vi "RH_Auto_with_Lockin_clear_3.vi"() -> ()   [LabVIEW 2019]
uses:
  <vilib>/Instr/_visa.llb/VISA Configure Serial Port (Instr).vi
  <vilib>/ptbypt/NI_PtbyPt.lvlib
panel:
  out "T Graph":cluster{"X":dbl[], "Y":dbl[]}[](graph) caption="XY Graph"
  in  "Ramp [K/min]":bool
  in  "Ramp Mode":bool
  in  "Lakeshore Termination Character":u8=10 format="%.0x"
  in  "Apply voltage":bool
  out "read buffer":string
  in  "Target [V]":string
  in  "start [V]":string
  in  "Keithley2400":refnum<visa-resource-name>="GPIB1::15::INSTR"
  out "Resistance [Ohm]":dbl=97.3586 format="%#_6f"
  out "Lockin y (V)":dbl=136.05
  out "Lockin x (V)":dbl=0.000139774
  in  "On:Delta  Off:Lock-in":bool=TRUE
  in  "I for Lockin [A]":dbl=5e-06 format="%#_6e"
  out "Lockin Y (V)":dbl=-136.536
  out "Lockin X (V)":dbl=0.000486793
  in  "Lockin SR830":refnum<visa-resource-name>="GPIB1::8::INSTR"
  in  "Main sorb T control":bool
  in  "Wait [min]":i32
  in  "LakeShore335 (for He3)":refnum<visa-resource-name>="COM4"
  in  "Temp control off":bool
  out "Sample  T [K]":dbl=1.4
  out "Waiting T-stability":bool caption="stabilizing"
  in  "Set Initial Field":bool
  in  "Field [T]":dbl
  in  "Period [s]":dbl=0.3 caption="Delay Time (s)"
  in  "Measure R-T":bool
  in  "Save R-T":bool
  out "R-T":cluster{"X":dbl[], "Y":dbl[]}[](graph) caption="XY Graph"
  out "Rate [K/min]":dbl=-2.426094015917322 format="%#_6f"
  in  "Reset":bool
  in  "Stop":bool
  in  "Pause off":bool
  in  "Compliance [V]":dbl=1.0 format="%#_6f"
  out "R-H":cluster{"X":dbl[], "Y":dbl[]}[](graph) caption="XY Graph"
  in  "Reset":bool
  in  "Folder":path=path "C:/User Data/Graham" caption="Filename"
  out "Filename Out":path=path "C:/User Data/Bart/CG014_1012_3.00K"
  in  "File name":string="CG017a_3uA"
  out "VTI [K]":dbl=3.087
  out "VTI [K]":dbl=84.053
  out "Sample Temp [K]":dbl=1.4
  out "Magnetic Field [T]":dbl=2.97271
  out "Delta reading [Ohm]":dbl
  out "Delta Reading [Ohm]":dbl=355.153687
  out "Sample Temp [K]":dbl=186.475
  in  "Abort Delta":bool
  in  "Arm Delta":bool
  in  "DELAY [sec]":dbl=0.002 format="%#_6e"
  in  "I-HIGH [A]":dbl=1e-05 format="%#_6e"
  in  "Measure R-H":bool
  in  "Rate [K/min]":dbl=10.0
  in  "Set Temp [K]":dbl=20.0
  in  "Set Temperature":bool
  out "Magnetic Field [T]":dbl
  in  "Rate [T/min]":dbl=0.5
  in  "Set Field [T]":dbl
  in  "Set Field":bool
  in  "Keithley":refnum<visa-resource-name>="GPIB1::20::INSTR"
  in  "Skip":bool
  in  "Wait T-stable [min]":i32=30
  in  "period (s)":dbl=0.5 min=0.0 max=1111.0 step=0.1
  in  "stop 2":bool caption="Pause"
  in  "Wait field stable [sec]":dbl=20.0
  in  "Magnet Power supply":refnum<visa-resource-name>="COM6"
  in  "Set Field [T]   Rate [T/min]":dbl[][](array[numeric])=[[0.0, 0.2], [-6.0, 0.2], [0.0, 0.2], [6.0, 0.2]]
  in  "Set Temp [K]":dbl[][](array[numeric])=[[10.0, 5.0], [0.0, 5.0], [0.0, 5.0], [0.0, 5.0], [0.0, 5.0]]
  in  "LakeShore340":refnum<visa-resource-name>="COM7"
  out "error out 3":errorcluster={"status"=FALSE, "code"=1073676294, "source"="VISA Read in RH_Auto_with_Lockin_clear.vi"}
  # "Manual control"
  # "R-H Auto Measurement"
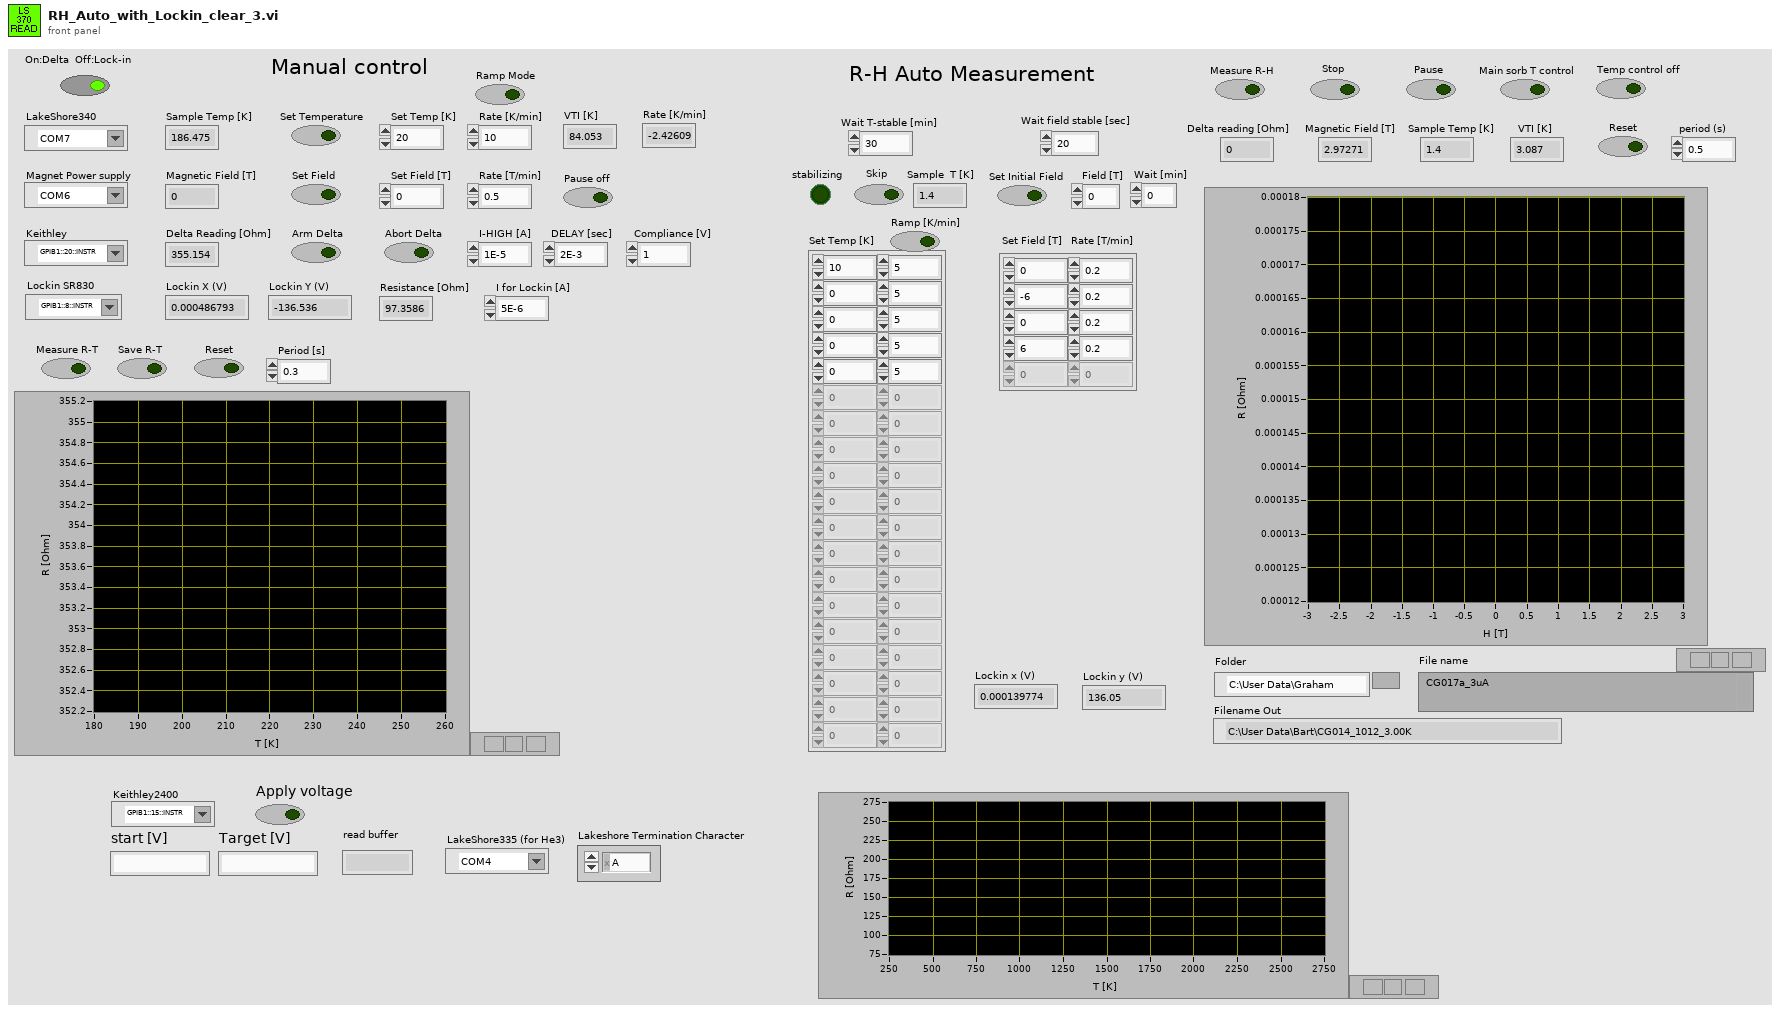
[diagram p1: front panel]
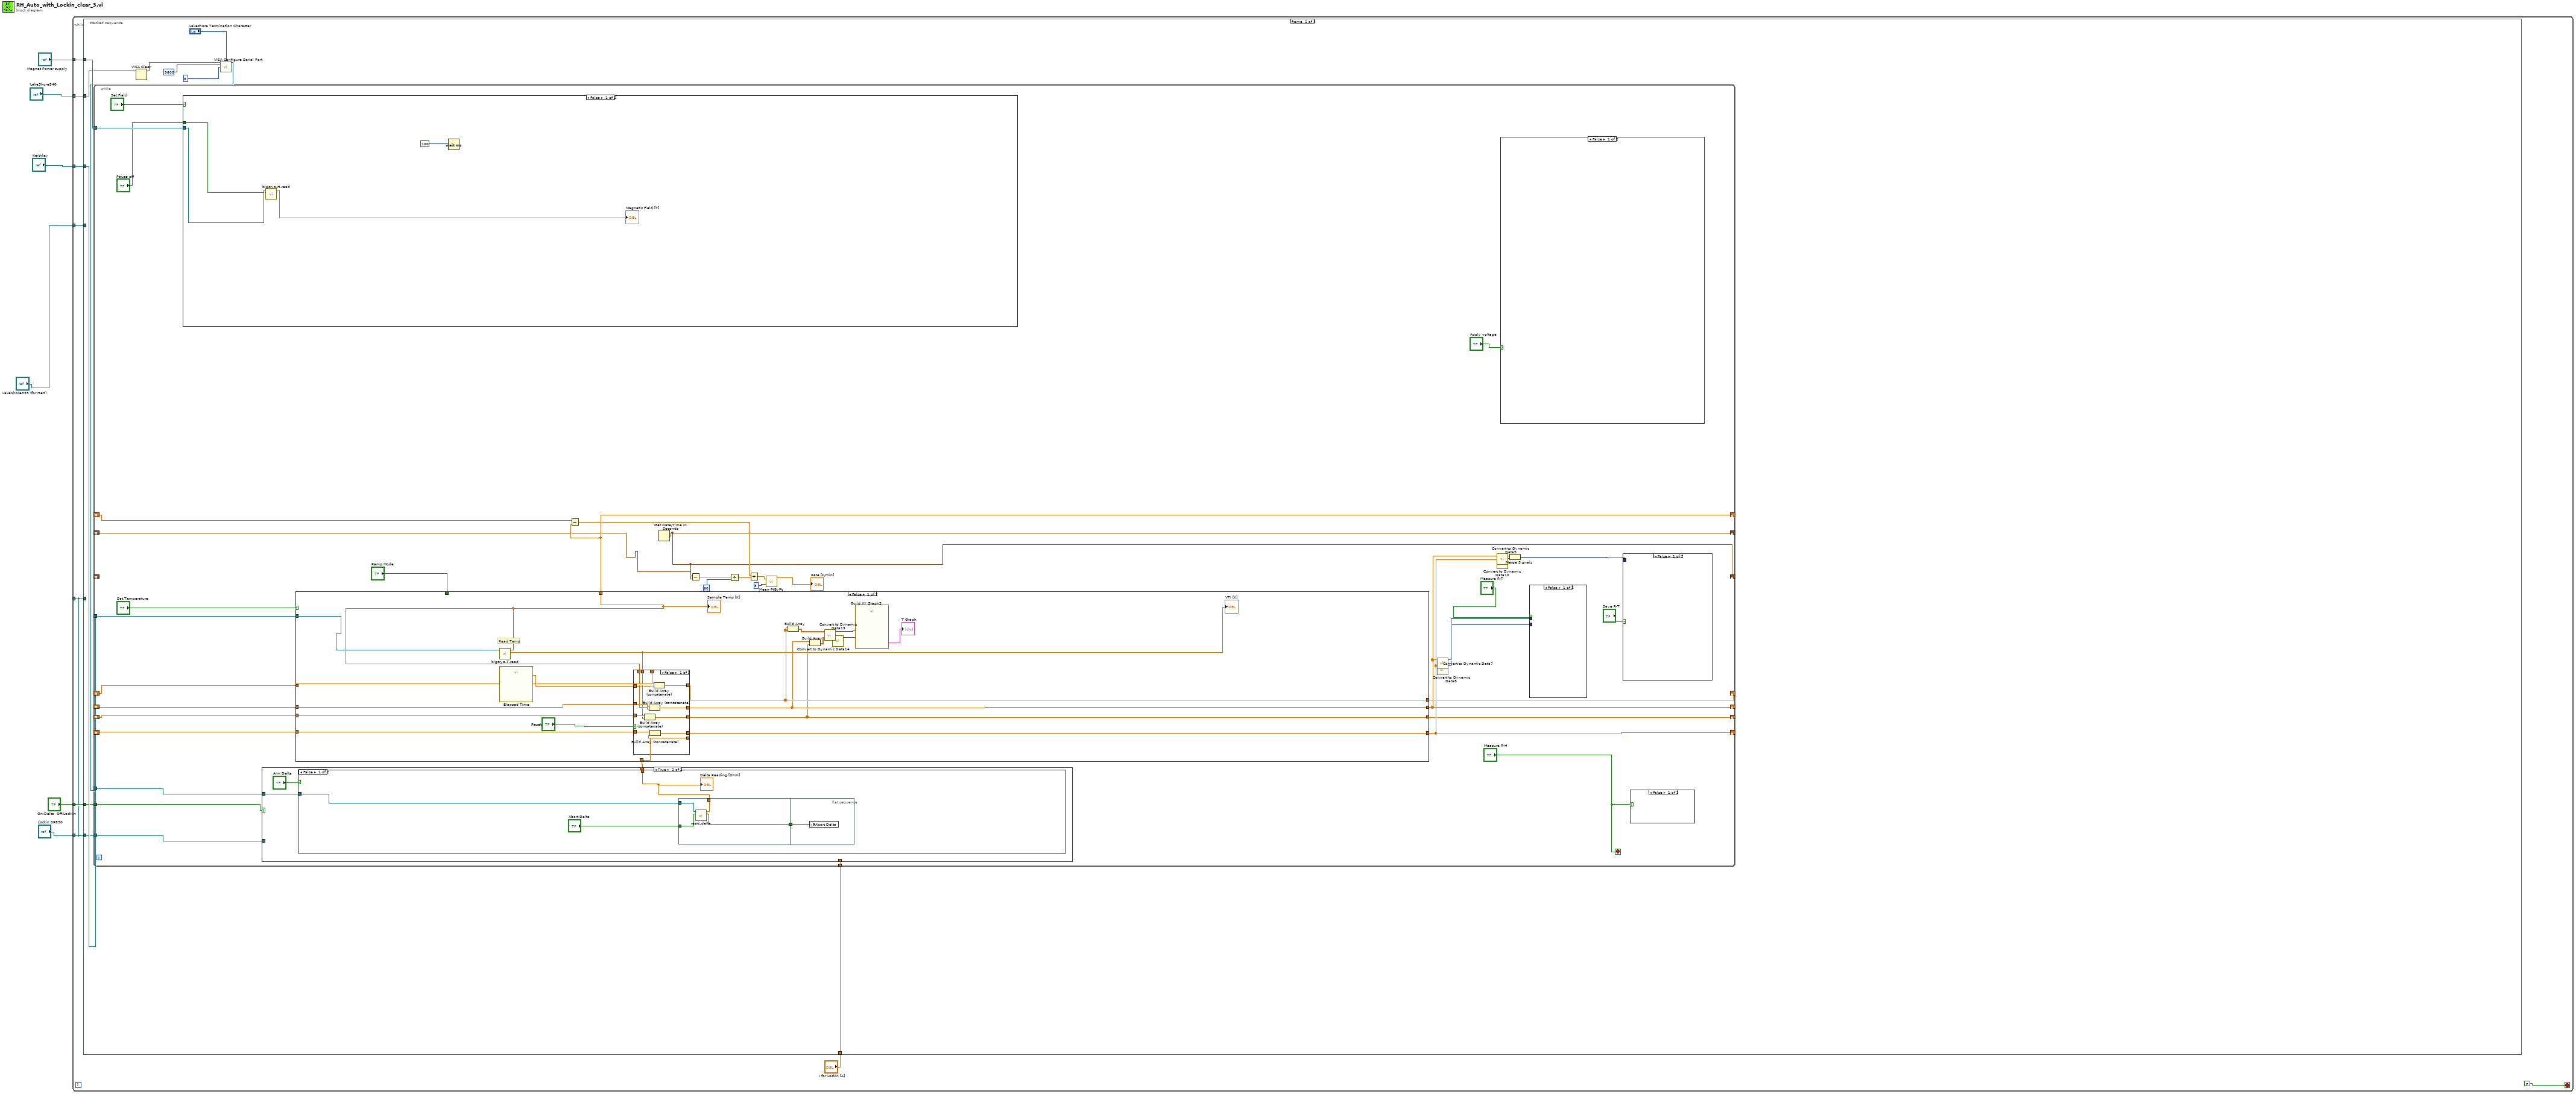
[diagram p0: block diagram]
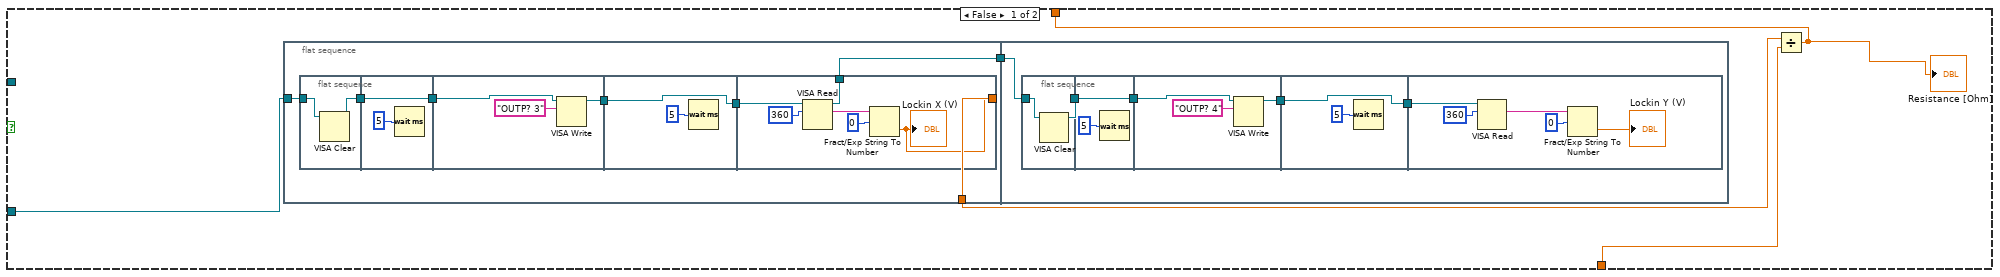
[diagram p2: hidden frame]
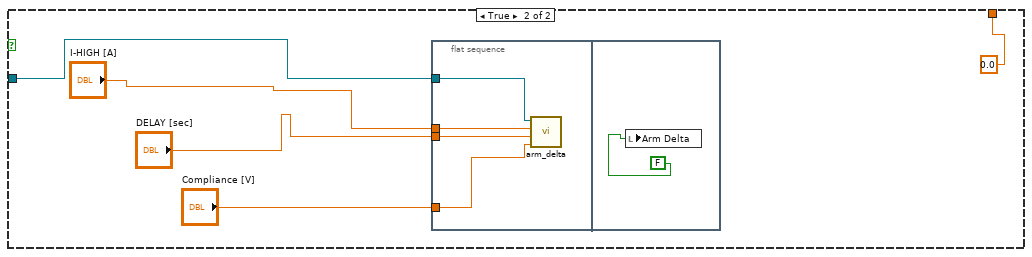
[diagram p3: hidden frame]
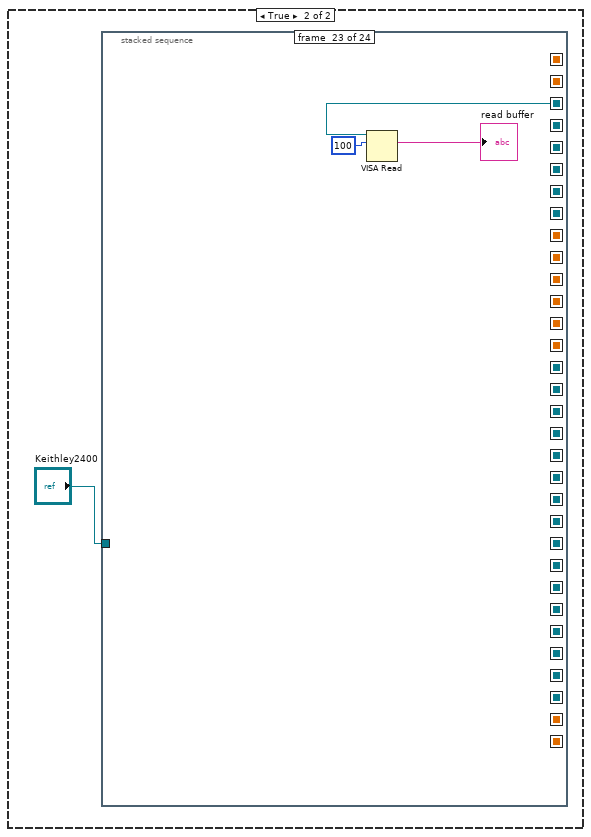
[diagram p4: hidden frame]
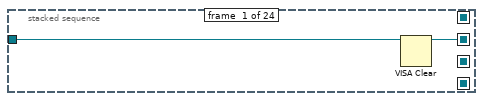
[diagram p5: hidden frame]
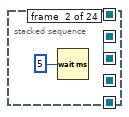
[diagram p6: hidden frame]
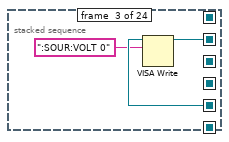
[diagram p7: hidden frame]
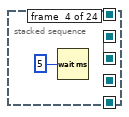
[diagram p8: hidden frame]
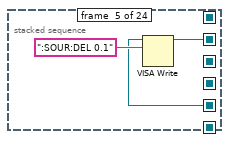
[diagram p9: hidden frame]
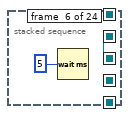
[diagram p10: hidden frame]
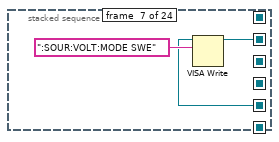
[diagram p11: hidden frame]
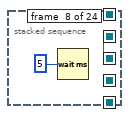
[diagram p12: hidden frame]
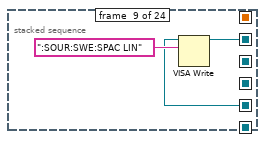
[diagram p13: hidden frame]
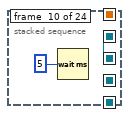
[diagram p14: hidden frame]
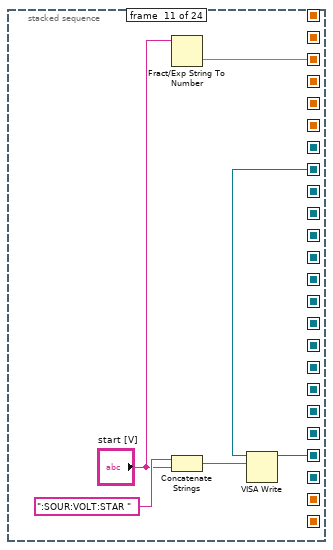
[diagram p15: hidden frame]
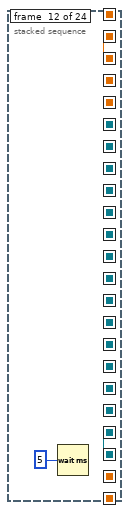
[diagram p16: hidden frame]
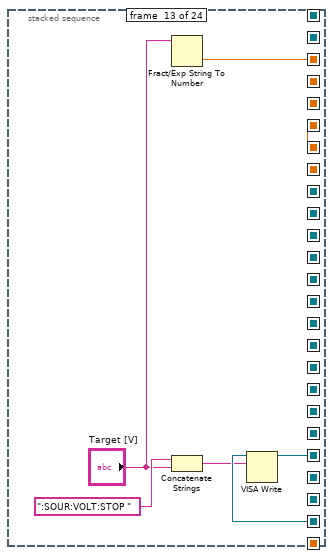
[diagram p17: hidden frame]
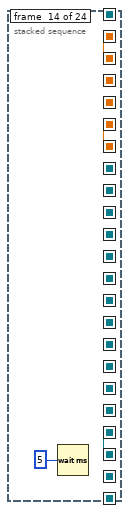
[diagram p18: hidden frame]
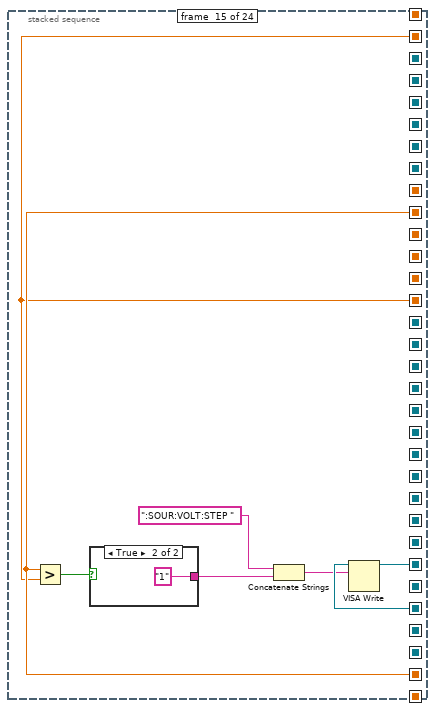
[diagram p19: hidden frame]
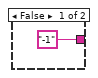
[diagram p20: hidden frame]
diagram:
  n1 = while {
    tunnel: "LakeShore340" -> [w14]
    tunnel: "Magnet Power supply" -> [w13]
    tunnel: "Keithley" -> [w12]
    tunnel: "LakeShore335 (for He3)" -> [w10]
    tunnel: "Lockin SR830" -> [w8]
    tunnel: "On:Delta  Off:Lock-in" -> [w9]
    tunnel: [w8] -> _
    stop <- FALSE stop-if-true
    n2 = stacked-sequence {
      tunnel: w14 -> [w15 w298 _]
      tunnel: w13 -> [w25 w297 w806]
      tunnel: w12 -> [w24 w296 _]
      tunnel: w10 -> [_ w294 _]
      tunnel: w8 -> [w23 _ _]
      tunnel: w9 -> [w22 w293 _]
      tunnel: w8 -> [_ w292 _]
      tunnel: "I for Lockin [A]" -> [w21 w291 _]
      frame #0 {
        n3 = VISA Clear(VISA resource name=w15) -> (VISA resource name out=w17:refnum<visa-resource-name>)  [unwired: 1 in, 1 out]
        n4 = call-poly "VISA Configure Serial Port"("VISA resource name"=w17, "termination char\n(0xA = '\\n' = LF)"="Lakeshore Termination Character", "baud rate (9600)"=9600, "data bits (8)"=8) -> ("VISA resource name out"=w16:refnum<visa-resource-name>)  [unwired: 10 in, 1 out]
        n5 = while {
          tunnel: w25 -> [w60]
          tunnel: w16 -> [w62]
          tunnel: w24 -> [w61]
          shift-right: [w48] -> _
          shift-left: _ -> [w43]
          shift-right: [w46] -> _
          shift-left: _ -> [w58]
          shift-right: [w40] -> _
          shift-left: _ -> [_]
          shift-right: [w56] -> _
          shift-left: _ -> [w57]
          shift-right: [w40] -> _
          shift-left: _ -> [w39]
          tunnel: w23 -> [w35]
          tunnel: w22 -> [w34]
          tunnel: w21 -> [w32]
          shift-right: [w29] -> _
          shift-left: _ -> [w28]
          shift-right: [w27] -> _
          shift-left: _ -> [w26]
          stop <- "Measure R-H" stop-if-true
          n6 = case shown="False" "Set Field" {
            tunnel: w60 -> [w284 w286]
            tunnel: "Pause off" -> [w283 _]
            frame False {
              n7 = call "bigcryo-H-read.vi"("Pause off"=w283, "Magnet Power supply"=w284) -> ("Magnetic Field [T]"=→"Magnetic Field [T]":dbl)  [unwired: 9 in]
              n8 = Wait (ms)(milliseconds to wait=100) -> ()  [unwired: 1 out]
            }
            frame True {
              n9 = flat-sequence {
                tunnel: w286 -> [w287]
                frame #0 {
                  n10 = call "bigcryo_H-control.vi"("Rate [T/min]"="Rate [T/min]", "Set Field [T]"="Set Field [T]", "Magnet Power supply"=w287) -> ()  [unwired: 9 in]
                }
                frame #1 {
                  n11 = local write "Set Field"(FALSE) -> ()
                }
              }
            }
          }
          n12 = case shown="True" w34 {
            tunnel: w61 -> [_ w113]
            tunnel: [w67 w111] -> w59
            tunnel: w35 -> [w68 _]
            tunnel: w32 -> [w65 _]
            frame False {
              n13 = flat-sequence {
                tunnel: [w74] -> w69
                tunnel: w68 -> [w73]
                tunnel: [w70] -> w66
                tunnel: w66 -> [w92]
                frame #0 {
                  n14 = flat-sequence {
                    tunnel: w73 -> [w78]
                    tunnel: [w77] -> w71
                    tunnel: [w80] -> w72
                    tunnel: w71 -> [w80]
                    tunnel: [w81] -> w76
                    tunnel: w72 -> [w83]
                    tunnel: [w84] -> w75
                    tunnel: w76 -> [w84]
                    tunnel: w75 -> [w89]
                    tunnel: [w87] -> w74
                    tunnel: [w86] -> w70
                    frame #0 {
                      n15 = VISA Clear(VISA resource name=w78) -> (VISA resource name out=w77:refnum<visa-resource-name>)  [unwired: 1 in, 1 out]
                    }
                    frame #1 {
                      n16 = Wait (ms)(milliseconds to wait=5) -> ()  [unwired: 1 out]
                    }
                    frame #2 {
                      n17 = VISA Write(VISA resource name=w83, write buffer="OUTP? 3" ("write buffer 2")) -> (VISA resource name out=w81:refnum<visa-resource-name>)  [unwired: 1 in, 2 out]
                    }
                    frame #3 {
                      n18 = Wait (ms)(milliseconds to wait=5) -> ()  [unwired: 1 out]
                    }
                    frame #4 {
                      n19 = VISA Read(VISA resource name=w89, byte count=u32 360) -> (VISA resource name out=w86:refnum<visa-resource-name>, read buffer=w88:string)  [unwired: 1 in, 2 out]
                      n20 = Fract/Exp String To Number(string=w88, offset=0) -> (number=w87:dbl)  [unwired: 3 out]
                      "Lockin X (V)" <- w87
                    }
                  }
                }
                frame #1 {
                  n21 = flat-sequence {
                    tunnel: w92 -> [w98]
                    tunnel: [w97] -> w93
                    tunnel: [w100] -> w94
                    tunnel: w93 -> [w100]
                    tunnel: [w101] -> w96
                    tunnel: w94 -> [w103]
                    tunnel: [w104] -> w95
                    tunnel: w96 -> [w104]
                    tunnel: w95 -> [w108]
                    frame #0 {
                      n22 = VISA Clear(VISA resource name=w98) -> (VISA resource name out=w97:refnum<visa-resource-name>)  [unwired: 1 in, 1 out]
                    }
                    frame #1 {
                      n23 = Wait (ms)(milliseconds to wait=5) -> ()  [unwired: 1 out]
                    }
                    frame #2 {
                      n24 = VISA Write(VISA resource name=w103, write buffer="OUTP? 4" ("write buffer 2")) -> (VISA resource name out=w101:refnum<visa-resource-name>)  [unwired: 1 in, 2 out]
                    }
                    frame #3 {
                      n25 = Wait (ms)(milliseconds to wait=5) -> ()  [unwired: 1 out]
                    }
                    frame #4 {
                      n26 = VISA Read(VISA resource name=w108, byte count=u32 360) -> (read buffer=w107:string)  [unwired: 1 in, 3 out]
                      n27 = Fract/Exp String To Number(string=w107, offset=0) -> (number=→"Lockin Y (V)":dbl)  [unwired: 3 out]
                    }
                  }
                }
              }
              n28 = Divide(x=w69, y=w65) -> (x/y=w67:dbl)
              "Resistance [Ohm]" <- w67
            }
            frame True {
              n29 = case shown="False" "Arm Delta" {
                tunnel: w113 -> [w116 w126]
                tunnel: [w117 0.0] -> w111
                frame False {
                  n30 = flat-sequence {
                    tunnel: [w121] -> w117
                    tunnel: w116 -> [w120]
                    tunnel: "Abort Delta" -> [w119]
                    tunnel: [w118] -> w114
                    tunnel: w114 -> [w122]
                    frame #0 {
                      n31 = call "read_delta.vi"("Abort Delta"=w119, "Keithley"=w120) -> ("aborted?"=w118:bool, "delta reading [ohm]"=w121:dbl)  [unwired: 8 in]
                    }
                    frame #1 {
                      n32 = local write "Abort Delta"(w122) -> ()
                    }
                  }
                  "Delta Reading [Ohm]" <- w117
                }
                frame True {
                  n33 = flat-sequence {
                    tunnel: w126 -> [w131]
                    tunnel: "I-HIGH [A]" -> [w130]
                    tunnel: "DELAY [sec]" -> [w129]
                    tunnel: "Compliance [V]" -> [w128]
                    frame #0 {
                      n34 = call "arm_delta.vi"("Compliance [V]"=w128, "DELAY [sec]"=w129, "I-HIGH [A]"=w130, "Keithley"=w131) -> ()  [unwired: 8 in]
                    }
                    frame #1 {
                      n35 = local write "Arm Delta"(FALSE ("Arm Delta")) -> ()
                    }
                  }
                }
              }
            }
          }
          n36 = case shown="False" "Set Temperature" {
            tunnel: w62 -> [w241 w273]
            tunnel: [w231 w276] -> w48
            tunnel: w43 -> [w246 w276]
            tunnel: w59 -> [w245 _]
            tunnel: [w244 w275] -> w46
            tunnel: w58 -> [w243 w275]
            tunnel: [w240 0.0] -> w56
            tunnel: "Ramp Mode" -> [_ w272]
            tunnel: [w230 w269] -> w29
            tunnel: w28 -> [w239 w269]
            tunnel: w26 -> [w236 w268]
            tunnel: [w232 w268] -> w27
            frame False {
              # "Read Temp"
              n37 = call "bigcryo-T-read.vi"("VISA resource name out"=w241) -> ("VTI Temp [K]"=w238:dbl, "Sample Temp [K]"=w240:dbl)  [unwired: 9 in]
              "Sample Temp [K]" <- w240
              "VTI [K]" <- w238
              n38 = call "Elapsed Time"() -> ("Elapsed Time (s)"=w237:dbl)  [unwired: 12 in, 7 out]
              n39 = case shown="False" "Reset" {
                tunnel: w240 -> [w258 _]
                tunnel: w246 -> [w257 _]
                tunnel: [w256 w262] -> w231
                tunnel: w245 -> [w255 _]
                tunnel: [w254 w261] -> w244
                tunnel: w243 -> [w253 _]
                tunnel: [w251 w260] -> w230
                tunnel: w239 -> [w252 _]
                tunnel: w238 -> [w250 _]
                tunnel: w237 -> [w249 _]
                tunnel: w236 -> [w248 _]
                tunnel: [w247 w259] -> w232
                frame False {
                  n40 = Build Array (concatenate)(w252, w250) -> (w251:dbl[])
                  n41 = Build Array (concatenate)(w257, w258) -> (w256:dbl[])
                  n42 = Build Array (concatenate)(w253, w255) -> (w254:dbl[])
                  n43 = Build Array (concatenate)(w248, w249) -> (w247:dbl[])
                }
                frame True {
                  n44 = stacked-sequence {
                    tunnel: [dbl[] [] _] -> w262
                    tunnel: [dbl[] [] _] -> w261
                    tunnel: [dbl[] [] _] -> w260
                    tunnel: [dbl[] [] _] -> w259
                    frame #0 {
                    }
                    frame #1 {
                      n45 = local write "Reset"(FALSE) -> ()
                    }
                  }
                }
              }
              n46 = Build Array(w232, w232) -> (w233:dbl[][])
              n47 = Build Array(w231, w230) -> (w229:dbl[][])
              n48 = call "Convert to Dynamic Data13"("2D Array"=w233) -> ("Dynamic Data Type"=w234:dynamicdata)  [unwired: 3 in]
              n49 = call "Convert to Dynamic Data14"("2D Array"=w229) -> ("Dynamic Data Type"=w228:dynamicdata)  [unwired: 3 in]
              n50 = call "Build XY Graph3"("Y Input"=w228, "X Input"=w234) -> ("XY Graph"=→"T Graph":cluster{"X":dbl[], "Y":dbl[]}[])  [unwired: 8 in, 1 out]
            }
            frame True {
              n51 = flat-sequence {
                tunnel: w273 -> [w280]
                tunnel: w272 -> [w279]
                tunnel: "Set Temp [K]" -> [w278]
                tunnel: "Rate [K/min]" -> [w277]
                frame #0 {
                  # "Control Temp"
                  n52 = call "bigcryo_T-control.vi"("Ramp Mode"=w279, "Rate  [K/min]"=w277, "VISA resource name out"=w280, "Set Sample Temp [K]"=w278) -> ()  [unwired: 12 in]
                }
                frame #1 {
                  n53 = local write "Set Temperature"(FALSE ("Set Temperature")) -> ()
                }
              }
            }
          }
          n54 = Subtract(x=w57, y=w56) -> (x-y=w52:dbl)
          n55 = Get Date/Time In Seconds() -> (seconds since 1Jan1904=w40:timestamp)
          n56 = Subtract(x=w39, y=w40) -> (x-y=w55:dbl)
          n57 = Divide(x=w55, y=60) -> (x/y=w53:dbl)
          n58 = Divide(x=w52, y=w53) -> (x/y=w37:dbl)
          n59 = call <vilib>:"Mean PtByPt.vi"("x"=w37, "sample length"=3) -> ("mean"=→"Rate [K/min]":dbl)  [unwired: 2 in, 1 out]
          n60 = call "Convert to Dynamic Data7"("Array"=w48) -> ("Dynamic Data Type"=w51:dynamicdata)  [unwired: 3 in]
          n61 = call "Convert to Dynamic Data8"("Array"=w46) -> ("Dynamic Data Type"=w50:dynamicdata)  [unwired: 3 in]
          n62 = call "Convert to Dynamic Data9"("Array"=w48) -> ("Dynamic Data Type"=w47:dynamicdata)  [unwired: 3 in]
          n63 = call "Convert to Dynamic Data10"("Array"=w46) -> ("Dynamic Data Type"=w45:dynamicdata)  [unwired: 3 in]
          n64 = case shown="False" "Apply voltage" {
            frame False {
            }
            frame True {
              n65 = stacked-sequence {
                seq-local: [w134 _ _ _ _ _ _ _ _ _ _ _ _ _ _ _ _ _ _ _ _ _ _ _] -> [_ w137 _ _ _ _ _ _ _ _ _ _ _ _ _ _ _ _ _ _ _ _ _ _]
                seq-local: [_ w137 _ _ _ _ _ _ _ _ _ _ _ _ _ _ _ _ _ _ _ _ _ _] -> [_ _ w140 _ _ _ _ _ _ _ _ _ _ _ _ _ _ _ _ _ _ _ _ _]
                seq-local: [_ _ w139 _ _ _ _ _ _ _ _ _ _ _ _ _ _ _ _ _ _ _ _ _] -> [_ _ _ w142 _ _ _ _ _ _ _ _ _ _ _ _ _ _ _ _ _ _ _ _]
                seq-local: [_ _ _ w142 _ _ _ _ _ _ _ _ _ _ _ _ _ _ _ _ _ _ _ _] -> [_ _ _ _ w144 _ _ _ _ _ _ _ _ _ _ _ _ _ _ _ _ _ _ _]
                seq-local: [_ _ _ _ w143 _ _ _ _ _ _ _ _ _ _ _ _ _ _ _ _ _ _ _] -> [_ _ _ _ _ w147 _ _ _ _ _ _ _ _ _ _ _ _ _ _ _ _ _ _]
                seq-local: [_ _ _ _ _ w147 _ _ _ _ _ _ _ _ _ _ _ _ _ _ _ _ _ _] -> [_ _ _ _ _ _ w149 _ _ _ _ _ _ _ _ _ _ _ _ _ _ _ _ _]
                seq-local: [_ _ _ _ _ _ w148 _ _ _ _ _ _ _ _ _ _ _ _ _ _ _ _ _] -> [_ _ _ _ _ _ _ w151 _ _ _ _ _ _ _ _ _ _ _ _ _ _ _ _]
                seq-local: [_ _ _ _ _ _ _ w151 _ _ _ _ _ _ _ _ _ _ _ _ _ _ _ _] -> [_ _ _ _ _ _ _ _ w154 _ _ _ _ _ _ _ _ _ _ _ _ _ _ _]
                seq-local: [_ _ _ _ _ _ _ _ w153 _ _ _ _ _ _ _ _ _ _ _ _ _ _ _] -> [_ _ _ _ _ _ _ _ _ w156 _ _ _ _ _ _ _ _ _ _ _ _ _ _]
                seq-local: [_ _ _ _ _ _ _ _ _ w156 _ _ _ _ _ _ _ _ _ _ _ _ _ _] -> [_ _ _ _ _ _ _ _ _ _ w163 _ _ _ _ _ _ _ _ _ _ _ _ _]
                seq-local: [_ _ _ _ _ _ _ _ _ _ w162 _ _ _ _ _ _ _ _ _ _ _ _ _] -> [_ _ _ _ _ _ _ _ _ _ _ w165 _ _ _ _ _ _ _ _ _ _ _ _]
                seq-local: [_ _ _ _ _ _ _ _ _ _ w158 _ _ _ _ _ _ _ _ _ _ _ _ _] -> [_ _ _ _ _ _ _ _ _ _ _ w164 _ _ _ _ _ _ _ _ _ _ _ _]
                seq-local: [_ _ _ _ _ _ _ _ _ _ _ w165 _ _ _ _ _ _ _ _ _ _ _ _] -> [_ _ _ _ _ _ _ _ _ _ _ _ w173 _ _ _ _ _ _ _ _ _ _ _]
                seq-local: [_ _ _ _ _ _ _ _ _ _ _ w164 _ _ _ _ _ _ _ _ _ _ _ _] -> [_ _ _ _ _ _ _ _ _ _ _ _ w167 _ _ _ _ _ _ _ _ _ _ _]
                seq-local: [_ _ _ _ _ _ _ _ _ _ _ _ w172 _ _ _ _ _ _ _ _ _ _ _] -> [_ _ _ _ _ _ _ _ _ _ _ _ _ w176 _ _ _ _ _ _ _ _ _ _]
                seq-local: [_ _ _ _ _ _ _ _ _ _ _ _ w168 _ _ _ _ _ _ _ _ _ _ _] -> [_ _ _ _ _ _ _ _ _ _ _ _ _ w175 _ _ _ _ _ _ _ _ _ _]
                seq-local: [_ _ _ _ _ _ _ _ _ _ _ _ w167 _ _ _ _ _ _ _ _ _ _ _] -> [_ _ _ _ _ _ _ _ _ _ _ _ _ w174 _ _ _ _ _ _ _ _ _ _]
                seq-local: [_ _ _ _ _ _ _ _ _ _ _ _ _ w176 _ _ _ _ _ _ _ _ _ _] -> [_ _ _ _ _ _ _ _ _ _ _ _ _ _ w185 _ _ _ _ _ _ _ _ _]
                seq-local: [_ _ _ _ _ _ _ _ _ _ _ _ _ w175 _ _ _ _ _ _ _ _ _ _] -> [_ _ _ _ _ _ _ _ _ _ _ _ _ _ w179 _ _ _ _ _ _ _ _ _]
                seq-local: [_ _ _ _ _ _ _ _ _ _ _ _ _ w174 _ _ _ _ _ _ _ _ _ _] -> [_ _ _ _ _ _ _ _ _ _ _ _ _ _ w178 _ _ _ _ _ _ _ _ _]
                seq-local: [_ _ _ _ _ _ _ _ _ _ _ _ _ _ w184 _ _ _ _ _ _ _ _ _] -> [_ _ _ _ _ _ _ _ _ _ _ _ _ _ _ w191 _ _ _ _ _ _ _ _]
                seq-local: [_ _ _ _ _ _ _ _ _ _ _ _ _ _ w179 _ _ _ _ _ _ _ _ _] -> [_ _ _ _ _ _ _ _ _ _ _ _ _ _ _ w189 _ _ _ _ _ _ _ _]
                seq-local: [_ _ _ _ _ _ _ _ _ _ _ _ _ _ w178 _ _ _ _ _ _ _ _ _] -> [_ _ _ _ _ _ _ _ _ _ _ _ _ _ _ w188 _ _ _ _ _ _ _ _]
                seq-local: [_ _ _ _ _ _ _ _ _ _ _ _ _ _ _ w191 _ _ _ _ _ _ _ _] -> [_ _ _ _ _ _ _ _ _ _ _ _ _ _ _ _ w202 _ _ _ _ _ _ _]
                seq-local: [_ _ _ _ _ _ _ _ _ _ _ _ _ _ _ w189 _ _ _ _ _ _ _ _] -> [_ _ _ _ _ _ _ _ _ _ _ _ _ _ _ _ w200 _ _ _ _ _ _ _]
                seq-local: [_ _ _ _ _ _ _ _ _ _ _ _ _ _ _ w188 _ _ _ _ _ _ _ _] -> [_ _ _ _ _ _ _ _ _ _ _ _ _ _ _ _ w199 _ _ _ _ _ _ _]
                seq-local: [_ _ _ _ _ _ _ _ _ _ _ _ _ _ _ _ w201 _ _ _ _ _ _ _] -> [_ _ _ _ _ _ _ _ _ _ _ _ _ _ _ _ _ w204 _ _ _ _ _ _]
                seq-local: [_ _ _ _ _ _ _ _ _ _ _ _ _ _ _ _ _ w204 _ _ _ _ _ _] -> [_ _ _ _ _ _ _ _ _ _ _ _ _ _ _ _ _ _ w206 _ _ _ _ _]
                seq-local: [_ _ _ _ _ _ _ _ _ _ _ _ _ _ _ _ _ _ w205 _ _ _ _ _] -> [_ _ _ _ _ _ _ _ _ _ _ _ _ _ _ _ _ _ _ w209 _ _ _ _]
                seq-local: [_ _ _ _ _ _ _ _ _ _ _ _ _ _ _ _ _ _ _ w209 _ _ _ _] -> [_ _ _ _ _ _ _ _ _ _ _ _ _ _ _ _ _ _ _ _ w211 _ _ _]
                seq-local: [_ _ _ _ _ _ _ _ _ _ _ _ _ _ _ _ _ _ _ _ w210 _ _ _] -> [_ _ _ _ _ _ _ _ _ _ _ _ _ _ _ _ _ _ _ _ _ w213 _ _]
                seq-local: [_ _ _ _ _ _ _ _ _ _ _ _ _ _ _ _ _ _ _ _ _ w213 _ _] -> [_ _ _ _ _ _ _ _ _ _ _ _ _ _ _ _ _ _ _ _ _ _ w217 _]
                tunnel: "Keithley2400" -> [w135 _ _ _ _ _ _ _ _ _ _ _ _ _ _ _ _ _ _ _ _ _ _ _]
                frame #0 {
                  n66 = VISA Clear(VISA resource name=w135) -> (VISA resource name out=w134:refnum<visa-resource-name>)  [unwired: 1 in, 1 out]
                }
                frame #1 {
                  n67 = Wait (ms)(milliseconds to wait=u32 5) -> ()  [unwired: 1 out]
                }
                frame #2 {
                  n68 = VISA Write(VISA resource name=w140, write buffer=":SOUR:VOLT 0" ("write buffer 2")) -> (VISA resource name out=w139:refnum<visa-resource-name>)  [unwired: 1 in, 2 out]
                }
                frame #3 {
                  n69 = Wait (ms)(milliseconds to wait=u32 5) -> ()  [unwired: 1 out]
                }
                frame #4 {
                  n70 = VISA Write(VISA resource name=w144, write buffer=":SOUR:DEL 0.1" ("write buffer 2")) -> (VISA resource name out=w143:refnum<visa-resource-name>)  [unwired: 1 in, 2 out]
                }
                frame #5 {
                  n71 = Wait (ms)(milliseconds to wait=u32 5) -> ()  [unwired: 1 out]
                }
                frame #6 {
                  n72 = VISA Write(VISA resource name=w149, write buffer=":SOUR:VOLT:MODE SWE" ("write buffer 2")) -> (VISA resource name out=w148:refnum<visa-resource-name>)  [unwired: 1 in, 2 out]
                }
                frame #7 {
                  n73 = Wait (ms)(milliseconds to wait=u32 5) -> ()  [unwired: 1 out]
                }
                frame #8 {
                  n74 = VISA Write(VISA resource name=w154, write buffer=":SOUR:SWE:SPAC LIN" ("write buffer 2")) -> (VISA resource name out=w153:refnum<visa-resource-name>)  [unwired: 1 in, 2 out]
                }
                frame #9 {
                  n75 = Wait (ms)(milliseconds to wait=u32 5) -> ()  [unwired: 1 out]
                }
                frame #10 {
                  n76 = Fract/Exp String To Number(string="start [V]") -> (number=w158:dbl)  [unwired: 3 in, 1 out]
                  n77 = Concatenate Strings(":SOUR:VOLT:STAR " ("write buffer 2"), "start [V]") -> (w160:string)
                  n78 = VISA Write(VISA resource name=w163, write buffer=w160) -> (VISA resource name out=w162:refnum<visa-resource-name>)  [unwired: 1 in, 2 out]
                }
                frame #11 {
                  n79 = Wait (ms)(milliseconds to wait=u32 5) -> ()  [unwired: 1 out]
                }
                frame #12 {
                  n80 = Fract/Exp String To Number(string="Target [V]") -> (number=w168:dbl)  [unwired: 3 in, 1 out]
                  n81 = Concatenate Strings(":SOUR:VOLT:STOP " ("write buffer 2"), "Target [V]") -> (w170:string)
                  n82 = VISA Write(VISA resource name=w173, write buffer=w170) -> (VISA resource name out=w172:refnum<visa-resource-name>)  [unwired: 1 in, 2 out]
                }
                frame #13 {
                  n83 = Wait (ms)(milliseconds to wait=u32 5) -> ()  [unwired: 1 out]
                }
                frame #14 {
                  n84 = Greater?(x=w179, y=w178) -> (0:w180:bool)
                  n85 = case shown="True" w180 {
                    tunnel: ["-1" "1"] -> w181
                    frame False {
                    }
                    frame True {
                    }
                  }
                  n86 = Concatenate Strings(":SOUR:VOLT:STEP " ("write buffer 2"), w181) -> (w183:string)
                  n87 = VISA Write(VISA resource name=w185, write buffer=w183) -> (VISA resource name out=w184:refnum<visa-resource-name>)  [unwired: 1 in, 2 out]
                }
                frame #15 {
                  n88 = Wait (ms)(milliseconds to wait=u32 5) -> ()  [unwired: 1 out]
                }
                frame #16 {
                  n89 = Subtract(x=w200, y=w199) -> (x-y=w198:dbl)
                  n90 = Absolute Value(x=w198) -> (abs(x)=w194:dbl)
                  n91 = Add(x=w194, y=1) -> (x+y=w192:dbl)
                  n92 = Number To Fractional String(number=w192) -> (F-format string=w196:string)  [unwired: 3 in]
                  n93 = Concatenate Strings(":TRIG:COUN " ("write buffer 2"), w196) -> (w197:string)
                  n94 = VISA Write(VISA resource name=w202, write buffer=w197) -> (VISA resource name out=w201:refnum<visa-resource-name>)  [unwired: 1 in, 2 out]
                }
                frame #17 {
                  n95 = Wait (ms)(milliseconds to wait=u32 5) -> ()  [unwired: 1 out]
                }
                frame #18 {
                  n96 = VISA Write(VISA resource name=w206, write buffer=":OUTP ON" ("write buffer 2")) -> (VISA resource name out=w205:refnum<visa-resource-name>)  [unwired: 1 in, 2 out]
                }
                frame #19 {
                  n97 = Wait (ms)(milliseconds to wait=u32 5) -> ()  [unwired: 1 out]
                }
                frame #20 {
                  n98 = VISA Write(VISA resource name=w211, write buffer=":READ?" ("write buffer 2")) -> (VISA resource name out=w210:refnum<visa-resource-name>)  [unwired: 1 in, 2 out]
                }
                frame #21 {
                  n99 = Wait (ms)(milliseconds to wait=u32 5) -> ()  [unwired: 1 out]
                }
                frame #22 {
                  n100 = VISA Read(VISA resource name=w217, byte count=u32 100) -> (read buffer=→"read buffer":string)  [unwired: 1 in, 3 out]
                }
                frame #23 {
                  n101 = local write "Apply voltage"(FALSE) -> ()
                }
              }
            }
          }
          n102 = Merge Signals(w47, w45) -> (w49:dynamicdata)
          n103 = case shown="False" "Measure R-T" {
            tunnel: w51 -> [_ w223]
            tunnel: w50 -> [_ w222]
            frame False {
            }
            frame True {
              n104 = call "Build XY Graph2"("Y Input"=w222, "X Input"=w223) -> ("XY Graph"=→"R-T":cluster{"X":dbl[], "Y":dbl[]}[])  [unwired: 8 in, 1 out]
              n105 = call "Time Delay16"("Delay Time (s)"="Period [s]") -> ()  [unwired: 10 in, 1 out]
            }
          }
          n106 = case shown="False" "Save R-T" {
            tunnel: w49 -> [_ w224]
            frame False {
            }
            frame True {
              n107 = flat-sequence {
                tunnel: w224 -> [w225]
                frame #0 {
                  n108 = call "Write To Measurement File2"("Signals"=w225, "Reset"=TRUE) -> ()  [unwired: 15 in, 3 out]
                }
                frame #1 {
                  n109 = local write "Save R-T"(FALSE) -> ()
                }
              }
            }
          }
          n110 = case shown="False" "Measure R-H" {
            frame False {
            }
            frame True {
              n111 = local write "Measure R-T"(FALSE) -> ()
            }
          }
        }
      }
      frame #1 {
        # "interlocks"
        n112 = Index Array(array="Set Temp [K]", index (col)=0) -> (element=w306:dbl[])  [unwired: 1 in]
        n113 = Index Array(array="Set Temp [K]", index (col)=1) -> (element=w313:dbl[])  [unwired: 1 in]
        n114 = Array Max & Min(array=w306) -> (max value=w300:dbl, min value=w309:dbl)  [unwired: 2 out]
        n115 = Array Max & Min(array=w313) -> (max value=w311:dbl)  [unwired: 3 out]
        n116 = Less?(x=w309, y=0) -> (x < y?=w310:bool)
        n117 = Greater?(x=w300, y=300) -> (0:w301:bool)
        n118 = Or(x=w301, y=w310) -> (x .or. y?=w314:bool)
        n119 = Greater?(x=w311, y=100) -> (0:w295:bool)
        n120 = call "Display Message to User2"("Enable"=w314) -> ("OK"=w315:bool)  [unwired: 9 in, 1 out]
        n121 = call "Display Message to User"("Enable"=w295) -> ("OK"=w302:bool)  [unwired: 9 in, 1 out]
        n122 = Or(x=w315, y=w302) -> (x .or. y?=w303:bool)
        n123 = while {
          tunnel: "Set Temp [K]" -> [w332]
          tunnel: w298 -> [w330]
          tunnel: w297 -> [w329]
          tunnel: w296 -> [w328]
          tunnel: w294 -> [w319]
          tunnel: w293 -> [w318]
          tunnel: w292 -> [w317]
          tunnel: w291 -> [w316]
          i -> [w331]
          stop <- w320 stop-if-true
          n124 = Matrix Size(0:w332) -> (1:w333:i32)  [unwired: 1 out]
          n125 = Less Or Equal?(x=w333, y=w331) -> (x <= y?=w323:bool)
          n126 = Index Array(array=w332, index (row)=w331) -> (element=w334:dbl[])  [unwired: 1 in]
          n127 = Index Array(array=w334, index=1) -> (element=w326:dbl)
          n128 = Index Array(array=w334, index=0) -> (element=w325:dbl)
          n129 = Multiply(x=w326, y=w325) -> (x*y=w327:dbl)
          n130 = Equal To 0?(x=w327) -> (x = 0?=w324:bool)
          n131 = Or(x=w324, y=w323) -> (x .or. y?=w322:bool)
          n132 = case shown="False" w322 {
            tunnel: w330 -> [w347 _]
            tunnel: w326 -> [w346 _]
            tunnel: w329 -> [w340 _]
            tunnel: w328 -> [w345 _]
            tunnel: w325 -> [w344 _]
            tunnel: [w343 FALSE ("Boolean")] -> w321
            tunnel: w319 -> [w341 _]
            tunnel: w318 -> [w339 _]
            tunnel: w317 -> [w338 _]
            tunnel: w316 -> [w337 _]
            frame False {
              n133 = stacked-sequence {
                tunnel: w347 -> [w348 w446]
                tunnel: w344 -> [w353 _]
                tunnel: w346 -> [w352 _]
                tunnel: w340 -> [w351 w445]
                tunnel: w345 -> [_ w444]
                tunnel: w344 -> [_ w443]
                tunnel: [_ w442] -> w343
                tunnel: "Field [T]" -> [w350 w441]
                tunnel: w341 -> [w349 _]
                tunnel: w339 -> [_ w440]
                tunnel: w338 -> [_ w439]
                tunnel: w337 -> [_ w438]
                frame #0 {
                  n134 = flat-sequence {
                    tunnel: w349 -> [w358]
                    tunnel: w353 -> [w357]
                    tunnel: w352 -> [w356]
                    tunnel: w348 -> [w354]
                    tunnel: w351 -> [w402]
                    tunnel: w350 -> [w400]
                    frame #0 {
                      n135 = case shown="False" "Temp control off" {
                        tunnel: w358 -> [w361 _]
                        tunnel: w357 -> [w364 _]
                        tunnel: w356 -> [w363 _]
                        tunnel: w354 -> [w359 _]
                        frame False {
                          n136 = case shown="False" "Main sorb T control" {
                            tunnel: w361 -> [_ w366]
                            tunnel: [w365 w366] -> w360
                            tunnel: w359 -> [w365 _]
                            frame False {
                            }
                            frame True {
                            }
                          }
                          n137 = stacked-sequence {
                            tunnel: w360 -> [_ w368 _ w373]
                            tunnel: w364 -> [_ w371 _ _]
                            tunnel: w363 -> [_ w370 _ _]
                            tunnel: "Main sorb T control" -> [_ _ _ w374]
                            frame #0 {
                              n138 = Wait (ms)(milliseconds to wait=u32 50) -> ()  [unwired: 1 out]
                            }
                            frame #1 {
                              n139 = call "bigcryo_T-control.vi"("Ramp Mode"="Ramp [K/min]", "Rate  [K/min]"=w370, "VISA resource name out"=w368, "Set Sample Temp [K]"=w371) -> ()  [unwired: 12 in]
                            }
                            frame #2 {
                              n140 = Wait (ms)(milliseconds to wait=u32 50) -> ()  [unwired: 1 out]
                            }
                            frame #3 {
                              n141 = flat-sequence {
                                tunnel: w374 -> [w376]
                                tunnel: w373 -> [w375]
                                frame #0 {
                                n142 = while {
                                tunnel: w376 -> [w379]
                                tunnel: w375 -> [w378]
                                i -> [w377]
                                stop <- w391 stop-if-true
                                n143 = case shown="False" w379 {
                                tunnel: ["KRDG? B" ("write buffer") "KRDG? A" ("write buffer")] -> w380
                                frame False {
                                }
                                frame True {
                                }
                                }
                                n144 = Concatenate Strings(w380, "\n") -> (w385:string)
                                n145 = VISA Write(VISA resource name=w378, write buffer=w385) -> (VISA resource name out=w384:refnum<visa-resource-name>)  [unwired: 1 in, 2 out]
                                n146 = Multiply(x="Wait T-stable [min]", y=60) -> (x*y=w390:i32)
                                n147 = Less?(x=w390, y=w377) -> (x < y?=w389:bool)
                                n148 = VISA Read(VISA resource name=w384, byte count=u32 100) -> (read buffer=w382:string)  [unwired: 1 in, 3 out]
                                n149 = Or(x=w389, y="Skip") -> (x .or. y?=w391:bool)
                                n150 = Wait (ms)(milliseconds to wait=1000) -> ()  [unwired: 1 out]
                                n151 = Fract/Exp String To Number(string=w382) -> (number=→"Sample  T [K]":dbl)  [unwired: 3 in, 1 out]
                                "Waiting T-stability" <- TRUE
                                }
                                }
                                frame #1 {
                                w397 = FALSE
                                n152 = local write "Skip"(w397) -> ()
                                n153 = local write "Reset"(TRUE) -> ()
                                n154 = local write "Waiting T-stability"(w397) -> ()
                                }
                              }
                            }
                          }
                        }
                        frame True {
                          n155 = local write "Reset"(TRUE) -> ()
                        }
                      }
                    }
                    frame #1 {
                      n156 = case shown="True" "Set Initial Field" {
                        tunnel: w402 -> [_ w405]
                        tunnel: w400 -> [_ w403]
                        frame False {
                        }
                        frame True {
                          n157 = stacked-sequence {
                            tunnel: w405 -> [w406 w409 _ w427 _ w432 _]
                            tunnel: 0.2 -> [_ _ _ w417 _ _ _]
                            tunnel: w403 -> [_ w407 _ _ _ _ _]
                            frame #0 {
                              n158 = VISA Clear(VISA resource name=w406) -> ()  [unwired: 1 in, 2 out]
                            }
                            frame #1 {
                              # "set set field"
                              n159 = Number To Fractional String(number=w407, width (-)=i16 6, precision (6)=i16 3) -> (F-format string=w412:string)  [unwired: 1 in]
                              n160 = Concatenate Strings("S [%][MID] " ("string"), w412) -> (w408:string)
                              n161 = Concatenate Strings(w408, "\r") -> (w411:string)
                              n162 = VISA Write(VISA resource name=w409, write buffer=w411) -> ()  [unwired: 1 in, 3 out]
                            }
                            frame #2 {
                              n163 = Wait (ms)(milliseconds to wait=500) -> ()  [unwired: 1 out]
                            }
                            frame #3 {
                              # "set rate"
                              n164 = Divide(x=w417, y=60.0) -> (x/y=w422:dbl)
                              n165 = Divide(x=w422, y=0.09797) -> (x/y=w420:dbl)
                              n166 = Number To Fractional String(number=w420, width (-)=i16 6, precision (6)=i16 3) -> (F-format string=w425:string)  [unwired: 1 in]
                              n167 = Concatenate Strings("S R " ("string"), w425) -> (w424:string)
                              n168 = Concatenate Strings(w424, "\r") -> (w429:string)
                              n169 = VISA Write(VISA resource name=w427, write buffer=w429) -> ()  [unwired: 1 in, 3 out]
                            }
                            frame #4 {
                              n170 = Wait (ms)(milliseconds to wait=500) -> ()  [unwired: 1 out]
                            }
                            frame #5 {
                              # "Go to set field"
                              n171 = Concatenate Strings("R [%][MID]" ("data"), "\r") -> (w434:string)
                              n172 = VISA Write(VISA resource name=w432, write buffer=w434) -> ()  [unwired: 1 in, 3 out]
                            }
                            frame #6 {
                              n173 = Multiply(x="Wait [min]", y=60000) -> (x*y=w437:i32)
                              n174 = Wait (ms)(milliseconds to wait=w437) -> ()  [unwired: 1 out]
                            }
                          }
                        }
                      }
                    }
                  }
                }
                frame #1 {
                  n175 = flat-sequence {
                    tunnel: [w462] -> w453
                    tunnel: [w463] -> w452
                    tunnel: ["Set Field [T]   Rate [T/min]"] -> w451
                    tunnel: w445 -> [w463]
                    tunnel: w444 -> [w462]
                    tunnel: w441 -> [w459]
                    tunnel: w453 -> [w487]
                    tunnel: [w487] -> w450
                    tunnel: [w486] -> w449
                    tunnel: w452 -> [w486]
                    tunnel: [w486] -> w448
                    tunnel: [w485] -> w447
                    tunnel: w451 -> [w485]
                    tunnel: w450 -> [w497]
                    tunnel: w449 -> [w496]
                    tunnel: w448 -> [w495]
                    tunnel: w447 -> [w494]
                    tunnel: w446 -> [w493]
                    tunnel: w443 -> [w492]
                    tunnel: [w491] -> w442
                    tunnel: w440 -> [w490]
                    tunnel: w439 -> [w489]
                    tunnel: w438 -> [w488]
                    frame #0 {
                      # "interlocks"
                      n176 = Index Array(array="Set Field [T]   Rate [T/min]", index (col)=0) -> (element=w471:dbl[])  [unwired: 1 in]
                      n177 = Array Max & Min(array=w471) -> (max value=w464:dbl, min value=w474:dbl)  [unwired: 2 out]
                      n178 = Index Array(array="Set Field [T]   Rate [T/min]", index (col)=1) -> (element=w482:dbl[])  [unwired: 1 in]
                      n179 = Array Max & Min(array=w482) -> (max value=w476:dbl, min value=w479:dbl)  [unwired: 2 out]
                      n180 = Greater?(x=w464, y=10) -> (0:w465:bool)
                      n181 = Less?(x=w474, y=-10) -> (x < y?=w475:bool)
                      n182 = Greater?(x=w459, y=10) -> (0:w458:bool)
                      n183 = Less?(x=w459, y=-10) -> (x < y?=w457:bool)
                      n184 = Or(x=w465, y=w475) -> (x .or. y?=w455:bool)
                      n185 = Or(x=w458, y=w457) -> (x .or. y?=w456:bool)
                      n186 = Greater?(x=w476, y=0.6) -> (0:w481:bool)
                      n187 = Less?(x=w479, y=-0.6) -> (x < y?=w480:bool)
                      n188 = Or(x=w456, y=w455) -> (x .or. y?=w454:bool)
                      n189 = call "Display Message to User4"("Enable"=w454) -> ("OK"=w484:bool)  [unwired: 9 in, 1 out]
                      n190 = Or(x=w481, y=w480) -> (x .or. y?=w483:bool)
                      n191 = call "Display Message to User3"("Enable"=w483) -> ("OK"=w466:bool)  [unwired: 9 in, 1 out]
                      n192 = Or(x=w484, y=w466) -> (x .or. y?=w467:bool)
                      n193 = Stop(stop? (T)=w467) -> ()
                    }
                    frame #1 {
                    }
                    frame #2 {
                      n194 = while {
                        tunnel: w497 -> [w518]
                        tunnel: w496 -> [w517]
                        tunnel: w495 -> [w512]
                        tunnel: w494 -> [w509]
                        tunnel: w493 -> [w508]
                        tunnel: w492 -> [w507]
                        tunnel: [w501] -> w491
                        tunnel: w490 -> [w500]
                        tunnel: w489 -> [w499]
                        tunnel: w488 -> [w498]
                        i -> [w513]
                        stop <- w502 stop-if-true
                        n195 = Matrix Size(0:w509) -> (1:w510:i32)  [unwired: 1 out]
                        n196 = Less Or Equal?(x=w510, y=w513) -> (x <= y?=w504:bool)
                        n197 = Index Array(array=w509, index (row)=w513) -> (element=w514:dbl[])  [unwired: 1 in]
                        n198 = Index Array(array=w514, index=1) -> (element=w506:dbl)
                        n199 = Equal To 0?(x=w506) -> (x = 0?=w505:bool)
                        n200 = Or(x=w505, y=w504) -> (x .or. y?=w503:bool)
                        n201 = Index Array(array=w514, index=0) -> (element=w511:dbl)
                        n202 = case shown="False" w503 {
                          tunnel: w518 -> [w529 _]
                          tunnel: w517 -> [w528 _]
                          tunnel: w506 -> [w527 _]
                          tunnel: w512 -> [w526 _]
                          tunnel: w511 -> [w525 _]
                          tunnel: w508 -> [w524 _]
                          tunnel: w507 -> [w523 _]
                          tunnel: [w522 FALSE] -> w501
                          tunnel: w500 -> [w521 _]
                          tunnel: w499 -> [w520 _]
                          tunnel: w498 -> [w519 _]
                          frame False {
                            n203 = stacked-sequence {
                              tunnel: w529 -> [_ w541]
                              tunnel: w528 -> [_ w540]
                              tunnel: w526 -> [w530 _]
                              tunnel: w525 -> [w531 w539]
                              tunnel: w527 -> [w532 _]
                              tunnel: w524 -> [_ w538]
                              tunnel: w523 -> [_ w537]
                              tunnel: [_ w536] -> w522
                              tunnel: w521 -> [_ w535]
                              tunnel: w520 -> [_ w534]
                              tunnel: w519 -> [_ w533]
                              frame #0 {
                                n204 = call "bigcryo_H-control.vi"("Rate [T/min]"=w532, "Set Field [T]"=w531, "Magnet Power supply"=w530) -> ()  [unwired: 9 in]
                              }
                              frame #1 {
                                n205 = while {
                                tunnel: w541 -> [w564]
                                tunnel: w540 -> [w565]
                                tunnel: w539 -> [w563]
                                tunnel: w538 -> [w561]
                                tunnel: w537 -> [w560]
                                shift-right: [w552] -> _
                                shift-left: _ -> [w559]
                                shift-right: [w555] -> _
                                shift-left: _ -> [w558]
                                shift-right: [w554] -> _
                                shift-left: _ -> [w557]
                                shift-right: [w553] -> _
                                shift-left: _ -> [w556]
                                tunnel: ["Stop"] -> w536
                                tunnel: w535 -> [w548]
                                tunnel: w534 -> [w547]
                                shift-right: [w546] -> _
                                shift-left: _ -> [w545]
                                shift-right: [w544] -> _
                                shift-left: _ -> [w543]
                                tunnel: w533 -> [w542]
                                stop <- w551 stop-if-true
                                n206 = stacked-sequence {
                                seq-local: [w574 _ _ _ _ _] -> [_ w639 _ _ _ _]
                                seq-local: [w573 _ _ _ _ _] -> [_ w638 _ _ _ _]
                                seq-local: [_ w640 _ _ _ _] -> [_ _ w660 _ _ _]
                                seq-local: [_ w630 _ _ _ _] -> [_ _ w659 _ _ _]
                                seq-local: [_ w638 _ _ _ _] -> [_ _ w651 _ _ _]
                                seq-local: [_ w629 _ _ _ _] -> [_ _ w649 _ _ _]
                                seq-local: [_ _ w660 _ _ _] -> [_ _ _ w703 _ _]
                                seq-local: [_ _ w659 _ _ _] -> [_ _ _ w702 _ _]
                                seq-local: [_ _ w650 _ _ _] -> [_ _ _ w701 _ _]
                                seq-local: [_ _ w649 _ _ _] -> [_ _ _ w694 _ _]
                                seq-local: [_ _ _ w703 _ _] -> [_ _ _ _ w768 _]
                                seq-local: [_ _ _ w702 _ _] -> [_ _ _ _ w761 _]
                                seq-local: [_ _ _ w701 _ _] -> [_ _ _ _ w762 _]
                                seq-local: [_ _ _ w701 _ _] -> [_ _ _ _ _ _]
                                seq-local: [_ _ _ w693 _ _] -> [_ _ _ _ w758 _]
                                seq-local: [w567 _ _ _ _ _] -> [_ _ _ _ w705 _]
                                seq-local: [w570 _ _ _ _ _] -> [_ _ _ _ w704 _]
                                tunnel: w564 -> [w575 _ _ _ _ _]
                                tunnel: w565 -> [w573 _ _ _ _ _]
                                tunnel: w561 -> [_ w631 _ _ _ _]
                                tunnel: w563 -> [_ _ w658 _ _ _]
                                tunnel: [_ _ w656 _ _ _] -> w562
                                tunnel: [_ _ _ _ w768 _] -> _
                                tunnel: w560 -> [_ _ _ _ w764 _]
                                tunnel: [_ _ _ _ w745 _] -> w552
                                tunnel: w559 -> [_ _ _ _ w757 _]
                                tunnel: [_ _ _ _ w739 _] -> w555
                                tunnel: w558 -> [_ _ _ _ w752 _]
                                tunnel: [_ _ _ _ w741 _] -> w554
                                tunnel: w557 -> [_ _ _ _ w711 _]
                                tunnel: [_ _ _ _ w742 _] -> w553
                                tunnel: w556 -> [_ _ _ _ w760 _]
                                tunnel: w548 -> [w572 w627 _ _ w706 _]
                                tunnel: w547 -> [w571 _ _ _ _ _]
                                tunnel: [_ _ _ _ w716 _] -> w546
                                tunnel: w545 -> [_ _ _ _ w710 _]
                                tunnel: [_ _ _ _ w714 _] -> w544
                                tunnel: w543 -> [_ _ _ _ w709 _]
                                tunnel: w542 -> [w569 _ _ _ _ _]
                                frame #0 {
                                n207 = case shown="False" w572 {
                                tunnel: w575 -> [w580 w625]
                                tunnel: [w580 w624] -> w574
                                tunnel: w571 -> [w576 _]
                                tunnel: [w579 w623] -> w568
                                tunnel: [w578 w623] -> w570
                                frame False {
                                n208 = flat-sequence {
                                tunnel: [w585] -> w579
                                tunnel: w576 -> [w584]
                                tunnel: [w583] -> w577
                                tunnel: [w606] -> w578
                                tunnel: w577 -> [w605]
                                frame #0 {
                                n209 = flat-sequence {
                                tunnel: w584 -> [w589]
                                tunnel: [w588] -> w582
                                tunnel: w582 -> [w591]
                                tunnel: [w591] -> w581
                                tunnel: [w592] -> w587
                                tunnel: w581 -> [w594]
                                tunnel: [w595] -> w586
                                tunnel: w587 -> [w595]
                                tunnel: w586 -> [w600]
                                tunnel: [w598] -> w585
                                tunnel: [w597] -> w583
                                frame #0 {
                                n210 = VISA Clear(VISA resource name=w589) -> (VISA resource name out=w588:refnum<visa-resource-name>)  [unwired: 1 in, 1 out]
                                }
                                frame #1 {
                                n211 = Wait (ms)(milliseconds to wait=5) -> ()  [unwired: 1 out]
                                }
                                frame #2 {
                                n212 = VISA Write(VISA resource name=w594, write buffer="OUTP? 3" ("write buffer 2")) -> (VISA resource name out=w592:refnum<visa-resource-name>)  [unwired: 1 in, 2 out]
                                }
                                frame #3 {
                                n213 = Wait (ms)(milliseconds to wait=5) -> ()  [unwired: 1 out]
                                }
                                frame #4 {
                                n214 = VISA Read(VISA resource name=w600, byte count=u32 360) -> (VISA resource name out=w597:refnum<visa-resource-name>, read buffer=w599:string)  [unwired: 1 in, 2 out]
                                n215 = Fract/Exp String To Number(string=w599, offset=0) -> (number=w598:dbl)  [unwired: 3 out]
                                "Lockin x (V)" <- w598
                                }
                                }
                                }
                                frame #1 {
                                n216 = flat-sequence {
                                tunnel: w605 -> [w610]
                                tunnel: [w609] -> w604
                                tunnel: w604 -> [w612]
                                tunnel: [w612] -> w603
                                tunnel: [w613] -> w608
                                tunnel: w603 -> [w615]
                                tunnel: [w616] -> w607
                                tunnel: w608 -> [w616]
                                tunnel: w607 -> [w620]
                                tunnel: [w618] -> w606
                                frame #0 {
                                n217 = VISA Clear(VISA resource name=w610) -> (VISA resource name out=w609:refnum<visa-resource-name>)  [unwired: 1 in, 1 out]
                                }
                                frame #1 {
                                n218 = Wait (ms)(milliseconds to wait=5) -> ()  [unwired: 1 out]
                                }
                                frame #2 {
                                n219 = VISA Write(VISA resource name=w615, write buffer="OUTP? 4" ("write buffer 2")) -> (VISA resource name out=w613:refnum<visa-resource-name>)  [unwired: 1 in, 2 out]
                                }
                                frame #3 {
                                n220 = Wait (ms)(milliseconds to wait=5) -> ()  [unwired: 1 out]
                                }
                                frame #4 {
                                n221 = VISA Read(VISA resource name=w620, byte count=u32 360) -> (read buffer=w619:string)  [unwired: 1 in, 3 out]
                                n222 = Fract/Exp String To Number(string=w619, offset=0) -> (number=w618:dbl)  [unwired: 3 out]
                                "Lockin y (V)" <- w618
                                }
                                }
                                }
                                }
                                }
                                frame True {
                                w623 = 0.0
                                n223 = VISA Write(VISA resource name=w625, write buffer="SENS:DATA:LATest?") -> (VISA resource name out=w624:refnum<visa-resource-name>)  [unwired: 1 in, 2 out]
                                }
                                }
                                n224 = Divide(x=w568, y=w569) -> (x/y=w567:dbl)
                                }
                                frame #1 {
                                n225 = Concatenate Strings("KRDG? A" ("write buffer"), "\n") -> (w636:string)
                                n226 = VISA Write(VISA resource name=w631, write buffer=w636) -> (VISA resource name out=w634:refnum<visa-resource-name>)  [unwired: 1 in, 2 out]
                                n227 = VISA Read(VISA resource name=w634, byte count=u32 100) -> (VISA resource name out=w629:refnum<visa-resource-name>, read buffer=w632:string)  [unwired: 1 in, 2 out]
                                n228 = case shown="True" w627 {
                                tunnel: [w642 w648] -> w640
                                tunnel: w639 -> [w642 w644]
                                tunnel: [0.0 w643] -> w630
                                frame False {
                                }
                                frame True {
                                n229 = VISA Read(VISA resource name=w644, byte count=u32 360) -> (VISA resource name out=w648:refnum<visa-resource-name>, read buffer=w646:string)  [unwired: 1 in, 2 out]
                                n230 = Fract/Exp String To Number(string=w646, offset=0) -> (number=w643:dbl)  [unwired: 3 out]
                                }
                                }
                                "Delta reading [Ohm]" <- w630
                                n231 = Fract/Exp String To Number(string=w632) -> (number=→"VTI [K]":dbl)  [unwired: 3 in, 1 out]
                                }
                                frame #2 {
                                # "Read Magnetic Field"
                                n232 = stacked-sequence {
                                seq-local: [w661 _ _ _ _ _ _ _] -> [_ w664 _ _ _ _ _ _]
                                seq-local: [_ w662 _ _ _ _ _ _] -> [_ _ w666 _ _ _ _ _]
                                seq-local: [_ w663 _ _ _ _ _ _] -> [_ _ w665 _ _ _ _ _]
                                seq-local: [_ _ w666 _ _ _ _ _] -> [_ _ _ w669 _ _ _ _]
                                seq-local: [_ _ w665 _ _ _ _ _] -> [_ _ _ w668 _ _ _ _]
                                seq-local: [_ _ _ w671 _ _ _ _] -> [_ _ _ _ w674 _ _ _]
                                seq-local: [_ _ _ w670 _ _ _ _] -> [_ _ _ _ w675 _ _ _]
                                seq-local: [_ _ _ _ w674 _ _ _] -> [_ _ _ _ _ w686 _ _]
                                seq-local: [_ _ _ _ w675 _ _ _] -> [_ _ _ _ _ w684 _ _]
                                seq-local: [_ _ _ _ _ w685 _ _] -> [_ _ _ _ _ _ _ w690]
                                seq-local: [_ _ _ _ _ w683 _ _] -> [_ _ _ _ _ _ _ w689]
                                tunnel: w651 -> [w661 _ _ _ _ _ _ _]
                                tunnel: [_ _ _ _ _ w676 _ _] -> w650
                                frame #0 {
                                }
                                frame #1 {
                                n233 = VISA Clear(VISA resource name=w664) -> (VISA resource name out=w662:refnum<visa-resource-name>, error out=w663:errorcluster)  [unwired: 1 in]
                                }
                                frame #2 {
                                n234 = call "Time Delay2"() -> ()  [unwired: 11 in, 1 out]
                                }
                                frame #3 {
                                n235 = Concatenate Strings("G O" ("Command"), "\r") -> (w672:string)
                                n236 = VISA Write(VISA resource name=w669, write buffer=w672, error in (no error)=w668) -> (VISA resource name out=w671:refnum<visa-resource-name>, error out=w670:errorcluster)  [unwired: 1 out]
                                }
                                frame #4 {
                                n237 = call "Time Delay3"() -> ()  [unwired: 11 in, 1 out]
                                }
                                frame #5 {
                                n238 = VISA Read(VISA resource name=w686, byte count=u32 30, error in (no error)=w684) -> (VISA resource name out=w685:refnum<visa-resource-name>, read buffer=w680:string, error out=w683:errorcluster)  [unwired: 1 out]
                                n239 = Match Pattern(string=w680, regular expression="OUTPUT:") -> (after substring=w678:string)  [unwired: 1 in, 3 out]
                                n240 = Match Pattern(string=w678, regular expression=" TESLA") -> (before substring=w677:string)  [unwired: 1 in, 3 out]
                                n241 = Fract/Exp String To Number(string=w677, offset=0) -> (number=w676:dbl)  [unwired: 2 in, 1 out]
                                }
                                frame #6 {
                                n242 = call "Time Delay12"() -> ()  [unwired: 11 in, 1 out]
                                }
                                frame #7 {
                                n243 = VISA Close(VISA resource name=w690, error in (no error)=w689) -> (error out=→"error out 3":errorcluster)
                                }
                                }
                                "Magnetic Field [T]" <- w650
                                n244 = Equal To 0?(x=w650) -> (x = 0?=w653:bool)
                                n245 = case shown="False" w653 {
                                tunnel: w650 -> [w691 _]
                                tunnel: [w691 1.1] -> w652
                                frame False {
                                }
                                frame True {
                                }
                                }
                                n246 = Subtract(x=w652, y=w658) -> (x-y=w654:dbl)
                                n247 = Absolute Value(x=w654) -> (abs(x)=w655:dbl)
                                n248 = Less?(x=w655, y=0.03) -> (x < y?=w656:bool)
                                }
                                frame #3 {
                                n249 = Concatenate Strings("KRDG? B" ("write buffer"), "\n") -> (w699:string)
                                n250 = VISA Write(VISA resource name=w694, write buffer=w699) -> (VISA resource name out=w697:refnum<visa-resource-name>)  [unwired: 1 in, 2 out]
                                n251 = VISA Read(VISA resource name=w697, byte count=u32 100) -> (read buffer=w695:string)  [unwired: 1 in, 3 out]
                                n252 = Fract/Exp String To Number(string=w695) -> (number=w693:dbl)  [unwired: 3 in, 1 out]
                                "Sample Temp [K]" <- w693
                                }
                                frame #4 {
                                # "Y(ohm)"
                                # "X(Ohm)"
                                # "Temp"
                                # "Delta"
                                # "Field"
                                # "Time"
                                n253 = case shown="False" w706 {
                                tunnel: [w780 w781] -> w712
                                tunnel: w711 -> [_ w781]
                                tunnel: w709 -> [w780 _]
                                frame False {
                                }
                                frame True {
                                }
                                }
                                n254 = call "Convert to Dynamic Data5"("Array"=w752) -> ("Dynamic Data Type"=w737:dynamicdata)  [unwired: 3 in]
                                n255 = call "Convert to Dynamic Data6"("Array"=w712) -> ("Dynamic Data Type"=w736:dynamicdata)  [unwired: 3 in]
                                n256 = Number To Fractional String(number=w764, precision (6)=2) -> (F-format string=w765:string)  [unwired: 2 in]
                                n257 = call "Build XY Graph"("Y Input"=w736, "X Input"=w737) -> ("XY Graph"=→"R-H":cluster{"X":dbl[], "Y":dbl[]}[])  [unwired: 8 in, 1 out]
                                n258 = Format Date/Time String(time format string (%c)="%H:%M:%S%3u") -> (date/time string=w719:string)  [unwired: 2 in]
                                n259 = Fract/Exp String To Number(string=w719) -> (number=w720:dbl)  [unwired: 3 in, 1 out]
                                n260 = Path To String(path="Folder") -> (string=w748:string)
                                n261 = Match Pattern(string=w719, regular expression=":") -> (after substring=w725:string)  [unwired: 1 in, 3 out]
                                n262 = Fract/Exp String To Number(string=w725) -> (number=w727:dbl)  [unwired: 3 in, 1 out]
                                n263 = Match Pattern(string=w725, regular expression=":") -> (after substring=w721:string)  [unwired: 1 in, 3 out]
                                n264 = Multiply(x=w720, y=3600.0) -> (x*y=w724:dbl)
                                n265 = Concatenate Strings(w748, "\\", "File name", "_" ("string"), w765, "K") -> (w763:string)
                                n266 = Fract/Exp String To Number(string=w721) -> (number=w718:dbl)  [unwired: 3 in, 1 out]
                                n267 = Multiply(x=w727, y=60.0) -> (x*y=w723:dbl)
                                n268 = Build Array (concatenate)(w752, w762) -> (w738:dbl[])
                                n269 = Build Array (concatenate)(w711, w761) -> (w740:dbl[])
                                n270 = Build Array (concatenate)(w760, w758) -> (w743:dbl[])
                                n271 = Add(x=w724, y=w723) -> (x+y=w722:dbl)
                                n272 = Add(x=w722, y=w718) -> (x+y=w717:dbl)
                                n273 = Build Array (concatenate)(w757, w717) -> (w744:dbl[])
                                n274 = String To Path(string=w763) -> (path=w747:path)
                                n275 = call "Convert to Dynamic Data"("Array"=w744) -> ("Dynamic Data Type"=w753:dynamicdata)  [unwired: 3 in]
                                n276 = call "Convert to Dynamic Data2"("Array"=w738) -> ("Dynamic Data Type"=w756:dynamicdata)  [unwired: 3 in]
                                n277 = call "Convert to Dynamic Data4"("Array"=w743) -> ("Dynamic Data Type"=w754:dynamicdata)  [unwired: 3 in]
                                n278 = call "Convert to Dynamic Data3"("Array"=w740) -> ("Dynamic Data Type"=w755:dynamicdata)  [unwired: 3 in]
                                n279 = call "Convert to Dynamic Data11"("Array"=w709) -> ("Dynamic Data Type"=w708:dynamicdata)  [unwired: 3 in]
                                n280 = call "Convert to Dynamic Data12"("Array"=w710) -> ("Dynamic Data Type"=w707:dynamicdata)  [unwired: 3 in]
                                n281 = case shown="False" w706 {
                                tunnel: [w769 w779] -> w759
                                tunnel: w756 -> [w772 w778]
                                tunnel: w755 -> [_ w777]
                                tunnel: w754 -> [w773 w776]
                                tunnel: w753 -> [w774 w775]
                                tunnel: w708 -> [w771 _]
                                tunnel: w707 -> [w770 _]
                                frame False {
                                n282 = Merge Signals(w772, w770, w771, w773, w774) -> (w769:dynamicdata)
                                }
                                frame True {
                                n283 = Merge Signals(w778, w777, w776, w775) -> (w779:dynamicdata)
                                }
                                }
                                n284 = call "Write To Measurement File"("Signals"=w759, "Reset"=TRUE, "Filename"=w747) -> ("Filename Out"=→"Filename Out":path)  [unwired: 14 in, 2 out]
                                n285 = case shown="False" "Reset" {
                                tunnel: [w787 dbl[] []] -> w745
                                tunnel: w744 -> [w787 _]
                                tunnel: w743 -> [w786 _]
                                tunnel: [w786 dbl[] []] -> w742
                                tunnel: [w785 dbl[] []] -> w741
                                tunnel: w740 -> [w785 _]
                                tunnel: [w784 dbl[] []] -> w739
                                tunnel: w738 -> [w784 _]
                                tunnel: w710 -> [w783 _]
                                tunnel: [w782 dbl[] []] -> w713
                                tunnel: [w783 dbl[] []] -> w715
                                tunnel: w709 -> [w782 _]
                                frame False {
                                }
                                frame True {
                                }
                                }
                                n286 = Build Array (concatenate)(w715, w704) -> (w716:dbl[])
                                n287 = Build Array (concatenate)(w713, w705) -> (w714:dbl[])
                                }
                                frame #5 {
                                n288 = local write "Reset"(FALSE) -> ()
                                }
                                }
                                n289 = while {
                                stop <- "stop 2" continue-if-true
                                }
                                n290 = call "Time Delay"("Delay Time (s)"="period (s)") -> ()  [unwired: 1 in, 10 out]
                                n291 = case shown="True" w562 {
                                tunnel: [FALSE w796] -> w550
                                frame False {
                                }
                                frame True {
                                n292 = flat-sequence {
                                tunnel: [TRUE] -> w796
                                frame #0 {
                                n293 = Multiply(x="Wait field stable [sec]", y=1000.0) -> (x*y=w797:dbl)
                                n294 = Wait (ms)(milliseconds to wait=w797) -> ()  [unwired: 1 out]
                                }
                                frame #1 {
                                }
                                }
                                }
                                }
                                n295 = Or(x="Stop", y=w550) -> (x .or. y?=w551:bool)
                                }
                              }
                            }
                          }
                          frame True {
                          }
                        }
                        n296 = Or(x=w503, y=w501) -> (x .or. y?=w502:bool)
                      }
                    }
                  }
                }
              }
            }
            frame True {
            }
          }
          n297 = Or(x=w322, y=w321) -> (x .or. y?=w320:bool)
        }
        n298 = Stop(stop? (T)=w303) -> ()
      }
      frame #2 {
        n299 = stacked-sequence {
          tunnel: w806 -> [w807 w810 _ w828 _ w833 _]
          tunnel: 0.1 -> [_ _ _ w818 _ _ _]
          tunnel: 0.0 -> [_ w808 _ _ _ _ _]
          frame #0 {
            n300 = VISA Clear(VISA resource name=w807) -> ()  [unwired: 1 in, 2 out]
          }
          frame #1 {
            # "set set field"
            n301 = Number To Fractional String(number=w808, width (-)=i16 6, precision (6)=i16 3) -> (F-format string=w813:string)  [unwired: 1 in]
            n302 = Concatenate Strings("S [%][MID] " ("string"), w813) -> (w809:string)
            n303 = Concatenate Strings(w809, "\r") -> (w812:string)
            n304 = VISA Write(VISA resource name=w810, write buffer=w812) -> ()  [unwired: 1 in, 3 out]
          }
          frame #2 {
            n305 = Wait (ms)(milliseconds to wait=500) -> ()  [unwired: 1 out]
          }
          frame #3 {
            # "set rate"
            n306 = Divide(x=w818, y=60.0) -> (x/y=w823:dbl)
            n307 = Divide(x=w823, y=0.09797) -> (x/y=w821:dbl)
            n308 = Number To Fractional String(number=w821, width (-)=i16 6, precision (6)=i16 3) -> (F-format string=w826:string)  [unwired: 1 in]
            n309 = Concatenate Strings("S R " ("string"), w826) -> (w825:string)
            n310 = Concatenate Strings(w825, "\r") -> (w830:string)
            n311 = VISA Write(VISA resource name=w828, write buffer=w830) -> ()  [unwired: 1 in, 3 out]
          }
          frame #4 {
            n312 = Wait (ms)(milliseconds to wait=500) -> ()  [unwired: 1 out]
          }
          frame #5 {
            # "Go to set field"
            n313 = Concatenate Strings("R [%][MID]" ("data"), "\r") -> (w835:string)
            n314 = VISA Write(VISA resource name=w833, write buffer=w835) -> ()  [unwired: 1 in, 3 out]
          }
          frame #6 {
            w836 = FALSE
            n315 = local write "Measure R-H"(w836) -> ()
            n316 = local write "Stop"(w836) -> ()
            n317 = Wait (ms)(milliseconds to wait=500) -> ()  [unwired: 1 out]
          }
        }
      }
    }
  }
